vi "Pulse.vi"(2 "error in":errorcluster, 3 "Data in":T1) -> (0 "error out":errorcluster, 1 "Data out":T1)   [LabVIEW 2017, in "Steps.lvlib"]
uses:
  Steps.lvlib
  Type_Defs/Data.ctl
  Type_Defs/Diagnostics.ctl
  Type_Defs/Systems.ctl
panel:
  out "Helical":dbl(graph)
  out "Toroidal":dbl(graph)
  in  "Step Back":bool
  in  "Continue":bool
  # "Verify that the pulse is correct."
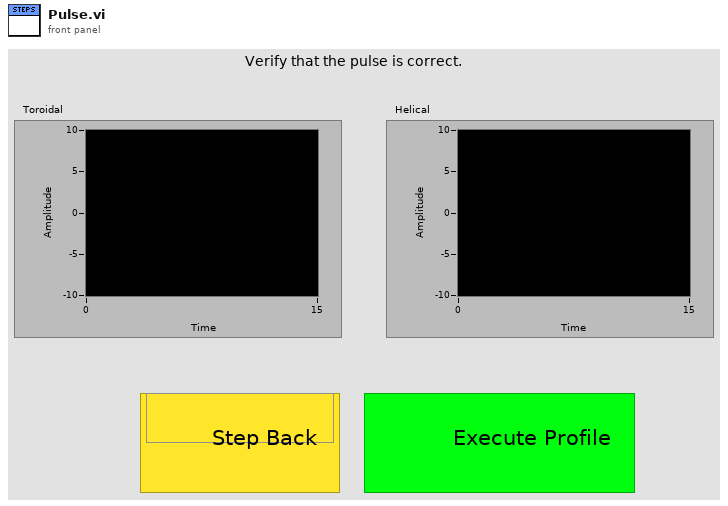
[diagram p1: front panel]
types:
  T1 = typedef "Data.ctl" = cluster{"User Name":string, "Experiment Number":i32, "Start Time":timestamp, "Data":dbl[], "Step Number":i32, "Step Instructions":string, "Diagnostics":T2, "Experiment Purpose":string, "Experiment State":enum16{"Off", "Setting Up", "Ready", "In Progress", "Shutting Down"}, "Systems":T3, "Vacuum Pressure":dbl, "Fieldpoints":cluster{"System Boolean Fieldpoints":cluster{"Compressed Air":refnum<k21>, "T-20kV Power Switch":refnum<k21>, "T-Rectifier":refnum<k21>, "Engage Interlock":refnum<k21>, "Ventilator":refnum<k21>, "Magnetron":refnum<k21>, "H-20kV Power Switch":refnum<k21>, "H-Rectifier":refnum<k21>, "Main Water Pump":refnum<k21>, "WEGA Water Pump":refnum<k21>, "Gas Inlet Valves":refnum<k21>}, "Step Fieldpoints":cluster{"Exhaust Ventillator":refnum<k21>, "Compressed Air":refnum<k21>, "Water Pressure":refnum<k21>, "Interlock":refnum<k21>, "Toroidal Power Supply 1":refnum<k21>, "Toroidal Power Supply 2":refnum<k21>, "Toroidal Rectifier":refnum<k21>, "Helical Power Supply":refnum<k21>, "Helical Rectifier":refnum<k21>, "6kW Magnetron Standby":refnum<k21>, "20kW Magnetron Standby":refnum<k21>}}, "Pressure History":cluster{"Seconds into Experiment":i32[], "Pressure Data":dbl[]}, "Time Computer Control":dbl[], "Toroidal Voltage Computer Control":dbl[], "Helical Voltage Computer Control":dbl[], "Toroidal Current":dbl[], "Toroidal Voltage":dbl[], "Toroidal Current Set Point":dbl[], "Helical Current Set Point":dbl[], "Helical Voltage":dbl[], "Helical Current":dbl[], "Experiment Folder":path, "Run Another Shot?":bool}
  T2 = typedef "Diagnostics.ctl" = cluster{"Langmuir Probe":bool, "Rogowski 1":bool, "Rogowski 2":bool, "Rogowski 3":bool, "B-dot 1":bool, "B-dot 2":bool}
  T3 = typedef "Systems.ctl" = cluster{"Compressed Air":bool, "T-20kV Power Switch":bool, "T-Rectifier":bool, "Engage Interlock":bool, "Ventilator":bool, "Magnetron":bool, "H-20kV Power Switch":bool, "H-Rectifier":bool, "Main Water Pump":bool, "WEGA Water Pump":bool, "Gas Inlet Valves":bool}
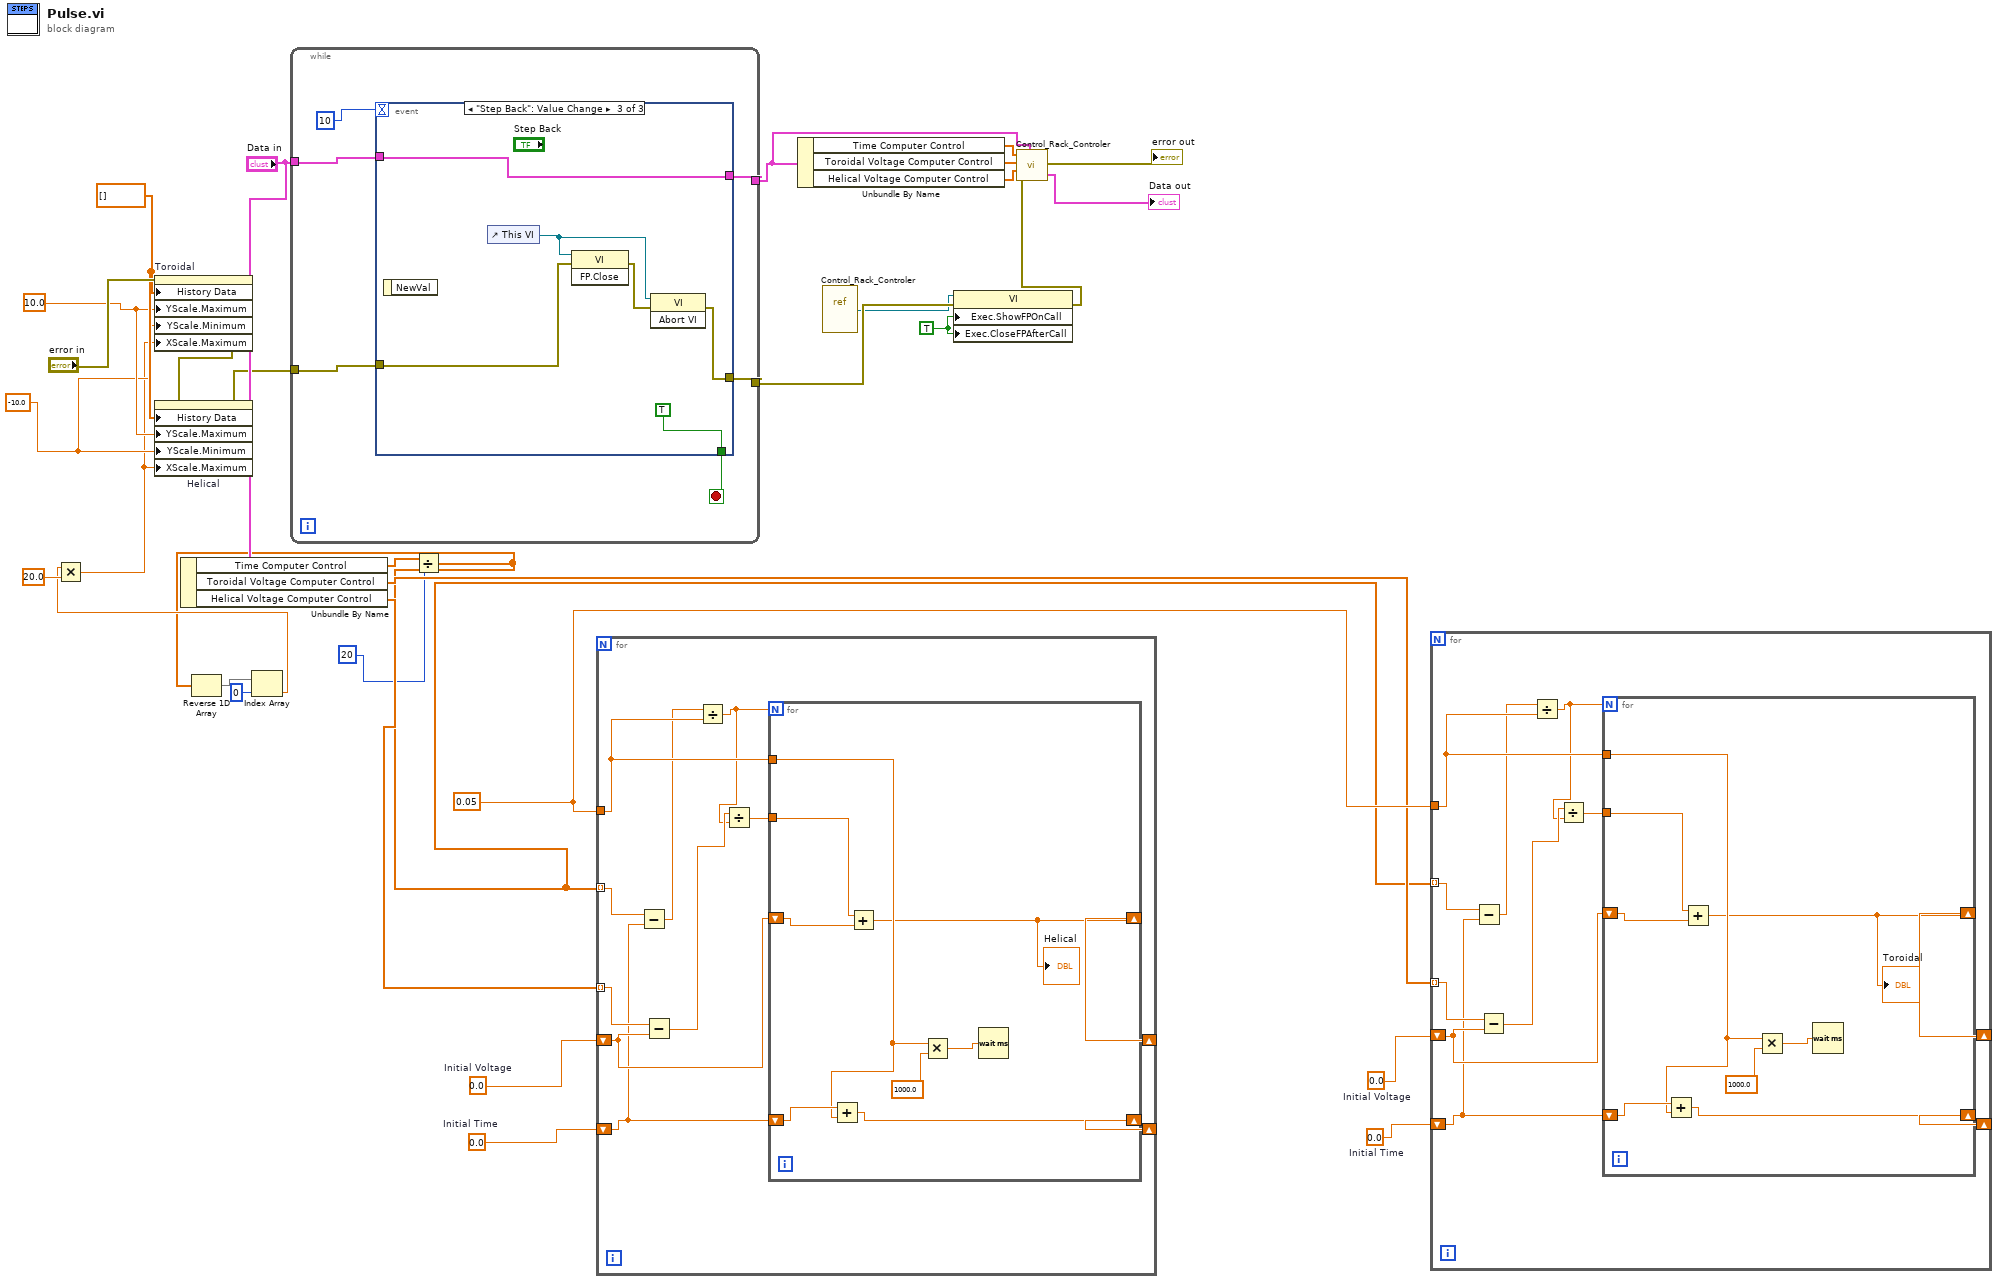
[diagram p0: block diagram]
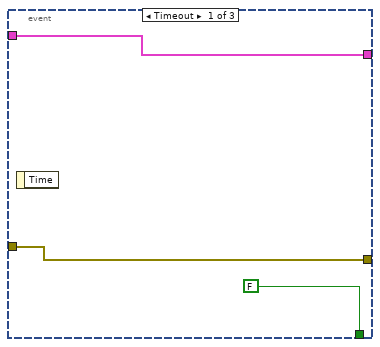
[diagram p2: hidden frame]
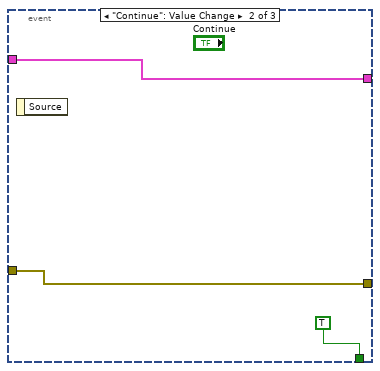
[diagram p3: hidden frame]
diagram:
  w7 = -10.0 ("Y Scale.Range:Maximum")
  w8 = 10.0 ("Y Scale.Range:Maximum")
  w11 = dbl[] [] ("History Data")
  w17 = 0.05 ("Timestep (in seconds, keep above 1/20s)")
  w19 = 0.0  # Initial Time
  w18 = 0.0  # Initial Voltage
  w20 = 0.0  # Initial Time
  w21 = 0.0  # Initial Voltage
  w26 = TRUE ("Execution:Show Front Panel On Call")
  n1 = Unbundle By Name("Data in") -> ("Time Computer Control"=w2:dbl[], "Toroidal Voltage Computer Control"=w15:dbl[], "Helical Voltage Computer Control"=w16:dbl[])
  n2 = Divide(x=w2, y=20 ("Time Computer Control")) -> (x/y=w3:dbl[])
  n3 = Reverse 1D Array(array=w3) -> (reversed array=w10:dbl[])
  n4 = Index Array(array=w10, index=0) -> (element=w5:dbl)
  n5 = Multiply(x=w5, y=20.0) -> (x*y=w4:dbl)
  n6 = property on="Toroidal" class="WFChart (strict)"(error in="error in", "History Data"=w11, "YScale.Maximum"=w8, "YScale.Minimum"=w7, "XScale.Maximum"=w4) -> (error out=w13:errorcluster)  [unwired: 1 in, 1 out]
  n7 = property on="Helical" class="WFChart (strict)"(error in=w13, "History Data"=w11, "YScale.Maximum"=w8, "YScale.Minimum"=w7, "XScale.Maximum"=w4) -> (error out=w12:errorcluster)  [unwired: 1 in, 1 out]
  n8 = while {
    tunnel: w12 -> [w38]
    tunnel: [w37] -> w25
    tunnel: [w35] -> w28
    tunnel: "Data in" -> [w34]
    stop <- w36 stop-if-true
    n9 = event shown="[2] \"Step Back\": Value Change" {
      selector: _ -> [_ _ _]
      dyn-events: _ -> [_ _ _]
      timeout: 10 -> [_ _ _]
      tunnel: w38 -> [w40 w44 w48]
      tunnel: [w40 w44 w45] -> w37
      tunnel: [FALSE TRUE TRUE] -> w36
      tunnel: [w39 w42 w49] -> w35
      tunnel: w34 -> [w39 w42 w49]
      event Timeout {
        n10 = event-data() -> ()  [unwired: 1 in, 1 out]
      }
      event "Continue": Value Change {
        n11 = event-data() -> ()  [unwired: 1 in, 1 out]
      }
      event "Step Back": Value Change {
        n12 = event-data() -> ()  [unwired: 1 in, 1 out]
        n13 = control-ref of="This VI"() -> (w47:refnum<vi>)
        n14 = invoke class="VI" method="FP.Close"(reference=w47, error in=w48) -> (error out=w46:errorcluster)  [unwired: 1 in, 2 out]
        n15 = invoke class="VI" method="Abort VI"(reference=w47, error in=w46) -> (error out=w45:errorcluster)  [unwired: 1 in, 2 out]
      }
    }
  }
  n16 = for {
    tunnel: w16 -> [w61] mode=indexing
    tunnel: w3 -> [w54] mode=indexing
    tunnel: w17 -> [w56]
    shift-right: [w57] -> _
    shift-left: w21 -> [w60]
    shift-right: [w55] -> _
    shift-left: w20 -> [w53]
    n17 = Subtract(x=w54, y=w53) -> (x-y=w52:dbl)
    n18 = Subtract(x=w61, y=w60) -> (x-y=w59:dbl)
    n19 = Divide(x=w52, y=w56) -> (x/y=w51:dbl)
    n20 = Divide(x=w59, y=w51) -> (x/y=w58:dbl)
    n21 = for {
      N: w51 -> [_]
      shift-right: [w62] -> w57
      shift-left: w60 -> [w69]
      tunnel: w58 -> [w68]
      tunnel: w56 -> [w65]
      shift-right: [w63] -> w55
      shift-left: w53 -> [w67]
      n22 = Add(x=w67, y=w65) -> (x+y=w63:dbl)
      n23 = Add(x=w68, y=w69) -> (x+y=w62:dbl)
      "Helical" <- w62
      n24 = Multiply(x=w65, y=1000.0) -> (x*y=w66:dbl)
      n25 = Wait (ms)(milliseconds to wait=w66) -> ()  [unwired: 1 out]
    }
  }
  n26 = Unbundle By Name(w28) -> ("Time Computer Control"=w31:dbl[], "Toroidal Voltage Computer Control"=w30:dbl[], "Helical Voltage Computer Control"=w29:dbl[])
  n27 = vi-ref "Control_Rack_Controler.vi"() -> (w23:refnum<vi>)
  n28 = property class="VI"(reference=w23, error in=w25, "Exec.ShowFPOnCall"=w26, "Exec.CloseFPAfterCall"=w26) -> (error out=w24:errorcluster)  [unwired: 1 out]
  n29 = call "Control_Rack_Controler.vi"("Times"=w31, "Voltages Toroidal (Keep below |10|)"=w30, "Voltages Helical (Keep below |10|)"=w29, "error out"=w24, "Data out 2"=w28) -> ("error out 2"=→"error out":errorcluster, "Data out"=→"Data out":T1)
  n30 = for {
    tunnel: w15 -> [w80] mode=indexing
    tunnel: w3 -> [w73] mode=indexing
    tunnel: w17 -> [w75]
    shift-right: [w76] -> _
    shift-left: w18 -> [w79]
    shift-right: [w74] -> _
    shift-left: w19 -> [w72]
    n31 = Subtract(x=w73, y=w72) -> (x-y=w71:dbl)
    n32 = Subtract(x=w80, y=w79) -> (x-y=w78:dbl)
    n33 = Divide(x=w71, y=w75) -> (x/y=w70:dbl)
    n34 = Divide(x=w78, y=w70) -> (x/y=w77:dbl)
    n35 = for {
      N: w70 -> [_]
      shift-right: [w81] -> w76
      shift-left: w79 -> [w88]
      tunnel: w77 -> [w87]
      tunnel: w75 -> [w84]
      shift-right: [w82] -> w74
      shift-left: w72 -> [w86]
      n36 = Add(x=w86, y=w84) -> (x+y=w82:dbl)
      n37 = Add(x=w87, y=w88) -> (x+y=w81:dbl)
      "Toroidal" <- w81
      n38 = Multiply(x=w84, y=1000.0) -> (x*y=w85:dbl)
      n39 = Wait (ms)(milliseconds to wait=w85) -> ()  [unwired: 1 out]
    }
  }
